vi "WaveformsWithNoise.vi"() -> ()   [LabVIEW 2015]
uses:
  <vilib>/Analysis/3filter.llb/Butterworth Filter (DBL).vi
  <vilib>/measure/madcrms.llb/Basic Averaged DC-RMS for 1 Chan.vi
  <vilib>/measure/NI_MABase.lvlib
  <vilib>/Analysis/NI_AALBase.lvlib
  <vilib>/measure/NI_MAPro.lvlib
panel:
  in  "Sampling Info":cluster{"Fs":dbl, "#s":dbl}={"Fs"=5000.0, "#s"=100.0} {"Fs" format="%.2p"}
  out "Lock-in Signal":waveform(dbl)(graph)
  out "RMS Chart":dbl(graph)
  out "Reference Signal":waveform(dbl)(graph)
  out "Input + Noise":waveform(dbl)(graph)
  out "RMS Out":dbl
  out "Response Time (s)":dbl
  out "Cuttoff Frequency (Hz)":dbl
  in  "Stop Button":bool
  in  "Noise Amplitude (V)":dbl
  in  "Slider_Offset":dbl(slide) scale=-5.0..5.0
  in  "Slide_Amp":dbl(slide) scale=0.0..5.0
  in  "Frequency (Hz)":dbl=100.0
  # "Amplitude (V)"
  # "Offset (V)"
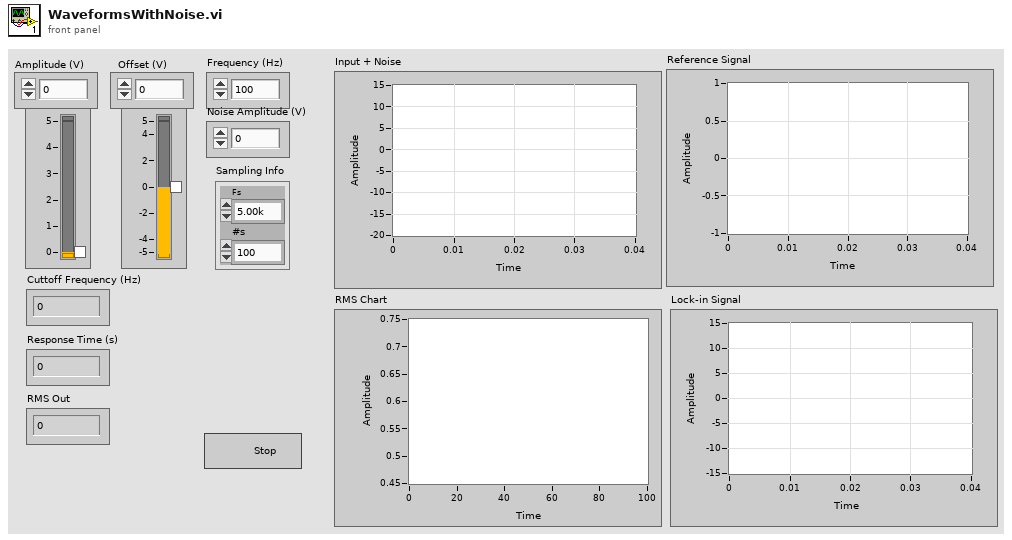
[diagram p1: front panel]
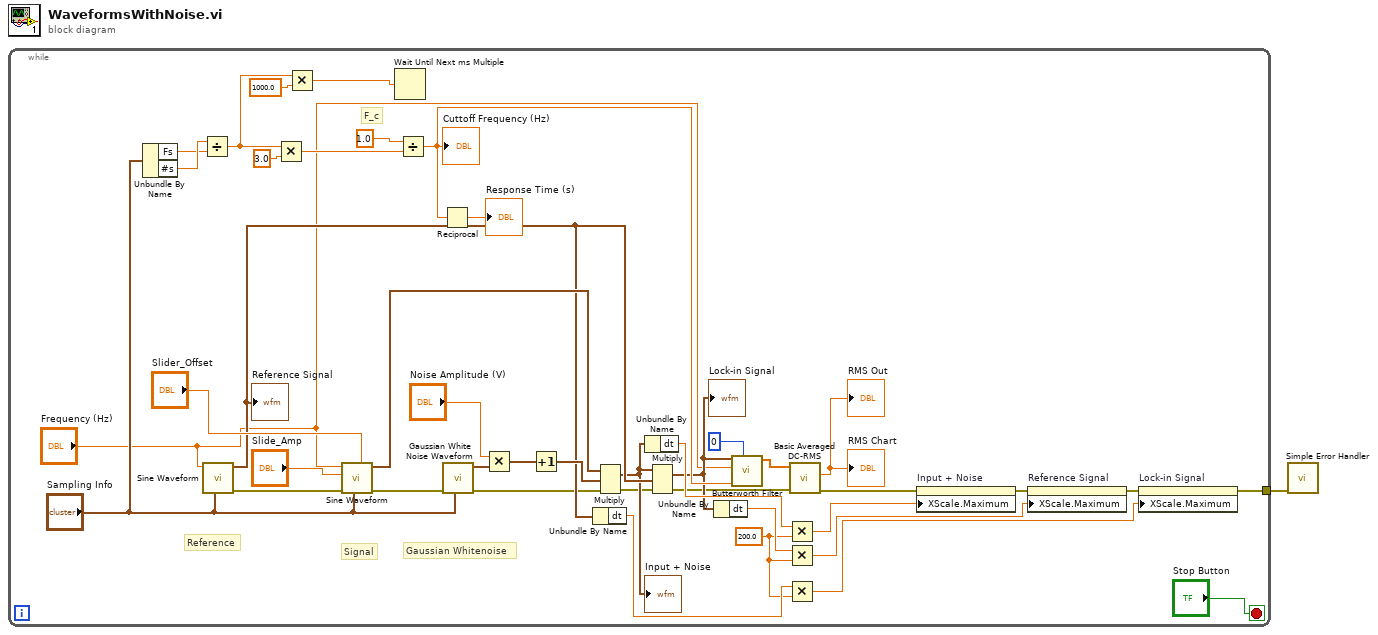
[diagram p0: block diagram]
diagram:
  n1 = while {
    tunnel: [w3] -> w1
    stop <- "Stop Button" stop-if-true
    w18 = 200.0 ("y")
    # "Gaussian Whitenoise"
    # "F_c"
    # "Reference"
    # "Signal"
    n2 = Unbundle By Name("Sampling Info") -> ("Fs"=w34:dbl, "#s"=w41:dbl)
    n3 = Divide(x=w41, y=w34) -> (x/y=w27:dbl)
    n4 = call <vilib>:"Sine Waveform.vi"("sampling info"="Sampling Info", "frequency"="Frequency (Hz)") -> ("error out"=w12:errorcluster, "signal out"=w24:waveform(dbl))  [unwired: 8 in]
    "Reference Signal" <- w24
    n5 = Multiply(x=w27, y=3.0) -> (x*y=w30:dbl)
    n6 = Multiply(x=w27, y=1000.0) -> (x*y=w29:dbl)
    n7 = call <vilib>:"Sine Waveform.vi"("offset"="Slider_Offset", "sampling info"="Sampling Info", "error in (no error)"=w12, "amplitude"="Slide_Amp", "frequency"="Frequency (Hz)") -> ("error out"=w11:errorcluster, "signal out"=w37:waveform(dbl))  [unwired: 5 in]
    n8 = Wait Until Next ms Multiple(millisecond multiple=w29) -> ()  [unwired: 1 out]
    n9 = Divide(x=1.0, y=w30) -> (x/y=w15:dbl)
    "Cuttoff Frequency (Hz)" <- w15
    n10 = Reciprocal(x=w15) -> (1/x=→"Response Time (s)":dbl)
    n11 = call <vilib>:"Gaussian White Noise Waveform.vi"("sampling info"="Sampling Info", "error in (no error)"=w11) -> ("error out"=w10:errorcluster, "signal out"=w40:waveform(dbl))  [unwired: 8 in]
    n12 = Multiply(x="Noise Amplitude (V)", y=w40) -> (x*y=w36:waveform(dbl))
    n13 = Increment(x=w36) -> (x+1=w35:waveform(dbl))
    n14 = Unbundle By Name(w24) -> ("dt"=w19:dbl)
    n15 = Multiply(1:w35, 2:w37, 4:w10) -> (0:w16:waveform(dbl), 3:w9:errorcluster)
    "Input + Noise" <- w16
    n16 = Unbundle By Name(w16) -> ("dt"=w21:dbl)
    n17 = Multiply(1:w24, 2:w16, 4:w9) -> (0:w13:waveform(dbl), 3:w7:errorcluster)
    "Lock-in Signal" <- w13
    n18 = Unbundle By Name(w13) -> ("dt"=w23:dbl)
    n19 = call-poly <vilib>:"Butterworth Filter.vi"("filter type"=0, "low cutoff freq: fl"=w15, "sampling freq: fs"="Frequency (Hz)", "X"=w13) -> ("Filtered X"=w14:dbl[])  [unwired: 4 in, 1 out]
    n20 = Multiply(x=w21, y=w18) -> (x*y=w20:dbl)
    n21 = Multiply(x=w23, y=w18) -> (x*y=w22:dbl)
    n22 = Multiply(x=w19, y=w18) -> (x*y=w17:dbl)
    n23 = call-poly <vilib>:"Basic Averaged DC-RMS.vi"("error in (no error)"=w7, "signal in"=w14) -> ("error out"=w6:errorcluster, "RMS value"=→"RMS Out" →"RMS Chart":dbl)  [unwired: 6 in, 2 out]
    n24 = property on="Input + Noise" class="WFGraph (strict)"(error in=w6, "XScale.Maximum"=w20) -> (error out=w5:errorcluster)  [unwired: 1 in, 1 out]
    n25 = property on="Reference Signal" class="WFGraph (strict)"(error in=w5, "XScale.Maximum"=w22) -> (error out=w4:errorcluster)  [unwired: 1 in, 1 out]
    n26 = property on="Lock-in Signal" class="WFGraph (strict)"(error in=w4, "XScale.Maximum"=w17) -> (error out=w3:errorcluster)  [unwired: 1 in, 1 out]
  }
  n27 = call <vilib>:"Simple Error Handler.vi"("error in (no error)"=w1) -> ()  [unwired: 4 in, 5 out]
